vi "Main.vi"() -> ()   [LabVIEW 2013]
doc: "This template is for the Queued Message Handler design pattern.\n\nThe Event Handling Loop generates messages based on user interface actions.\n\nThe Message Handling Loop processes messages generated by the Event Handling Loop, or by other messages. The messages are string values, so new messages can be added easily to the Message Cases case structure in the Message Handling Loop. Each message cluster can also provide an optional value for Message Data, which is a variant that can be converted to whatever message-specific data is required."
uses:
  <vilib>/vision/Image Controls.llb/IMAQ Image.ctl
  Message Passing/MsgQ Loops enum.ctl
  Image Processing/Mask ROI FG Enum.ctl
  System Status/Status FG Enum.ctl
  Globals/Average Sector Data.vi
  controls/UI Data.ctl
  Message Queue/Message Queue.lvlib
  User Event - Stop/User Event - Stop.lvlib
  Image Processing/Image Processing.lvlib
  Common/State Machines/State Machine Lib.lvlib
  Message Passing/Main MsgQ.lvlib
  Common/GUI/GUI.lvlib
  <vilib>/rvi/interface/nirviReadWriteControl/nirviReadWriteControl.xnode
  FGs/FPGA_Reference.ctl
  FPGA Bitfiles/8-Tap-No-DRAM.lvbitx
  <vilib>/rvi/errors/niLvFpgaMergeErrorWithErrorCode.vi
  NiFpgaLv.dll
  <vilib>/rvi/errors/niLvFpgaAdjustHostInterfaceError.vi
panel:
  out "Analysis Ticks":u32
  out "Accumulate Ticks":u32
  out "FPGA Display Image":T1(plugin-control)
  out "Right Wingbeat Avg Graph":u8[](graph)
  in  "Start Serial Server":bool=TRUE
  out "Left Wingbeat Avg Graph":u8[](graph)
  in  "Stop Charts":bool
  in  "Wing ROIs":T2
  out "FPGA image info":T5={"Image Type"=0, "Unit"=enum."Undefined", "X Resolution"=2040, "Y Resolution"=1088, "X Step"=1.0, "Y Step"=1.0, "Image Name"="Image"} {"Image Type" items=["Grayscale (U8)", "Grayscale (I16)", "Grayscale (SGL)", "Complex (CSG)", "RGB (U32)", "HSL (U32)", "RGB (U64)", "Grayscale (U16)"]}
  in  "Stream?":bool
  out "FPGA Image":T1
  in  "Test Visual Response":bool
  in  "Test FPGA":bool
  out "Status Update":string="VI Stopped"
  in  "Define Mask":bool
  in  "Acquire Image":bool
  in  "Stop":bool
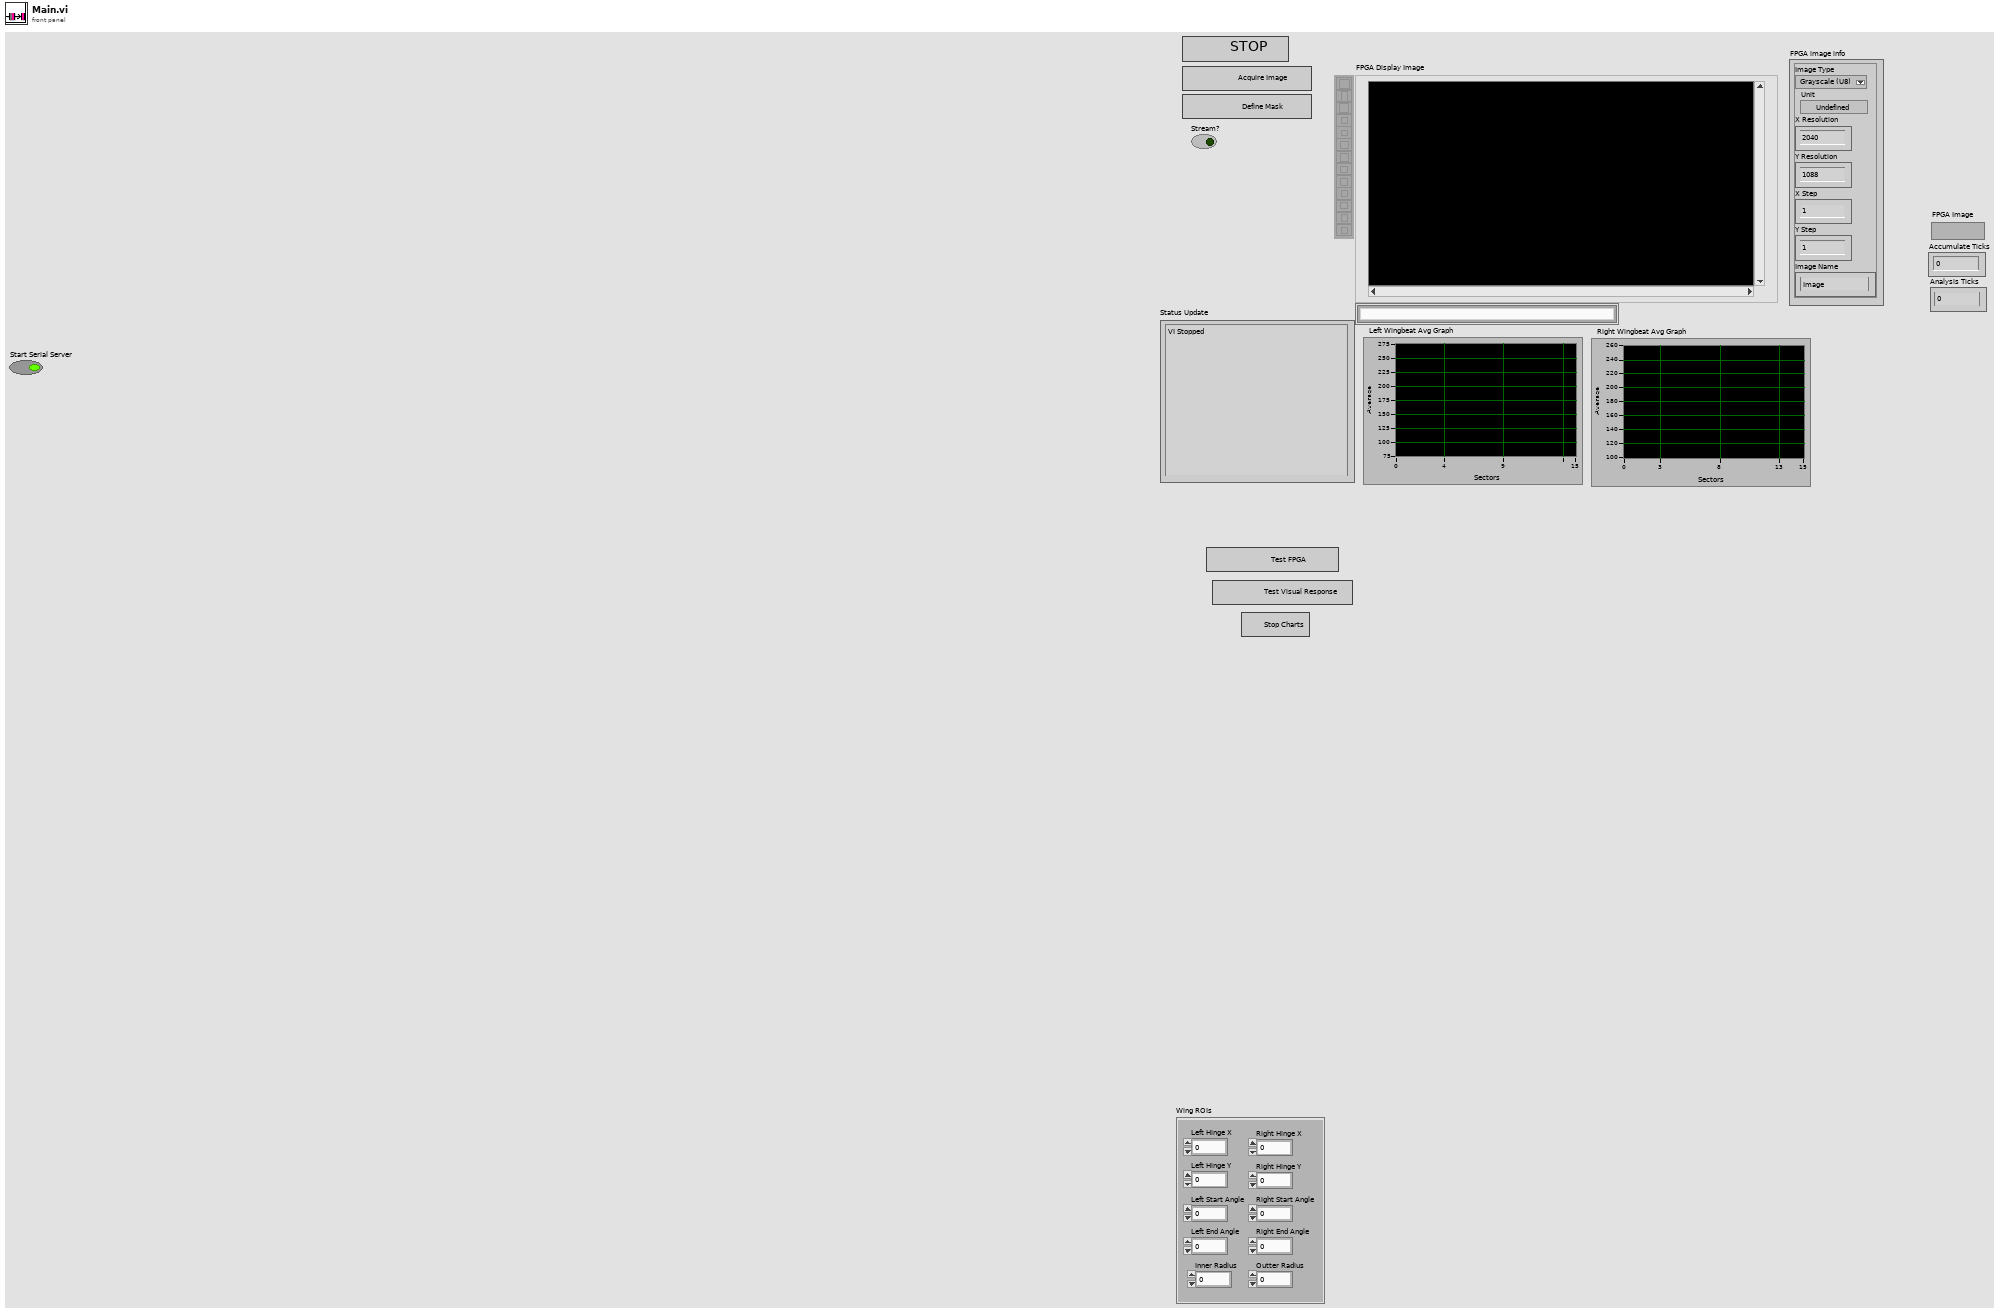
[diagram p1: front panel]
types:
  T1 = typedef "IMAQ Image.ctl" = refnum<image>
  T2 = cluster{"Left Hinge X":u16, "Left Hinge Y":u16, "Inner Radius":u16, "Outter Radius":u16, "Right Hinge X":u16, "Right Hinge Y":u16, "Right Start Angle":i16, "Right End Angle":i16, "Left Start Angle":i16, "Left End Angle":i16}
  T3 = typedef "Image Type" = u32
  T4 = typedef "Image Unit" = enum32{"Undefined", "Angström", "Micrometer", "Millimeter", "Centimeter", "Meter", "Kilometer", "Microinch", "Inch", "Feet", "Nautical miles", "Standard miles", "Steps"}
  T5 = cluster{"Image Type":T3, "Unit":T4, "X Resolution":i32, "Y Resolution":i32, "X Step":sgl, "Y Step":sgl, "Image Name":string}
  T6 = typedef "State Machine Lib.lvlib/STATE cluster.ctl" = cluster{"State":string, "Parameters":variant}
  T7 = typedef "Main MsgQ.lvlib/MsgQ Loops enum.ctl" = enum16{"User Interface", "Image Acq"}
  T8 = typedef "Status FG Enum.ctl" = enum16{"Reset", "Read", "Write"}
  T9 = typedef "Mask ROI FG Enum.ctl" = enum16{"Read", "Write"}
  T10 = typedef "FPGA_Reference.ctl" = refnum<k20>
  T11 = typedef "Mask ROI Cluster.ctl" = cluster{"left annulus":T12, "right annulus":T12, "Threshold Range":cluster{"Lower value":dbl, "Upper value":dbl}, "[Avg BG]":u8[], "Number of Sectors":u8, "Left ROI":T13, "Right ROI":T13, "Left Start Angle Duty Cycle":fxp<+,8,0>, "Left End Angle Duty Cycle":fxp<+,8,0>, "Right End Angle Duty Cycle":fxp<+,8,0>, "Right Start Angle Duty Cycle":fxp<+,8,0>, "[Sector ROIs]":T13[]}
  T12 = typedef "IMAQ Circle" = cluster{"Center X":i32, "Center Y":i32, "Inner Radius":i32, "Outer Radius":i32, "Start Angle":dbl, "End Angle":dbl}
  T13 = typedef "ROI Descriptor" = cluster{"Global Rectangle":i32[], "Contours":cluster{"ID":enum32{"External", "Internal"}, "Type":u32, "Coordinates":i32[]}[]}
  T14 = typedef "UI Data.ctl" = cluster{"Boolean <Replace Me>":bool, "Initial Message":string, "Numeric <Replace Me>":dbl, "Acquire Image Ref":refnum<vi>, "Define Mask Ref":refnum<vi>, "Status Update Ref":refnum<vi>, "Stop Button Ref":refnum<vi>, "FPGA Image":T1, "Processed Image":T1, "Left Annulus":cluster{"Center X":i32, "Center Y":i32, "Inner Radius":i32, "Outer Radius":i32, "Start Angle":dbl, "End Angle":dbl}, "Right Annulus":cluster{"Center X":i32, "Center Y":i32, "Inner Radius":i32, "Outer Radius":i32, "Start Angle":dbl, "End Angle":dbl}}
  T15 = typedef "Message Queue.lvlib/All Message Queues.ctl" = cluster{"UI":refnum<queue>}
  T16 = cluster{"Center X":i32, "Center Y":i32, "Inner Radius":i32, "Outer Radius":i32, "Start Angle":dbl, "End Angle":dbl}
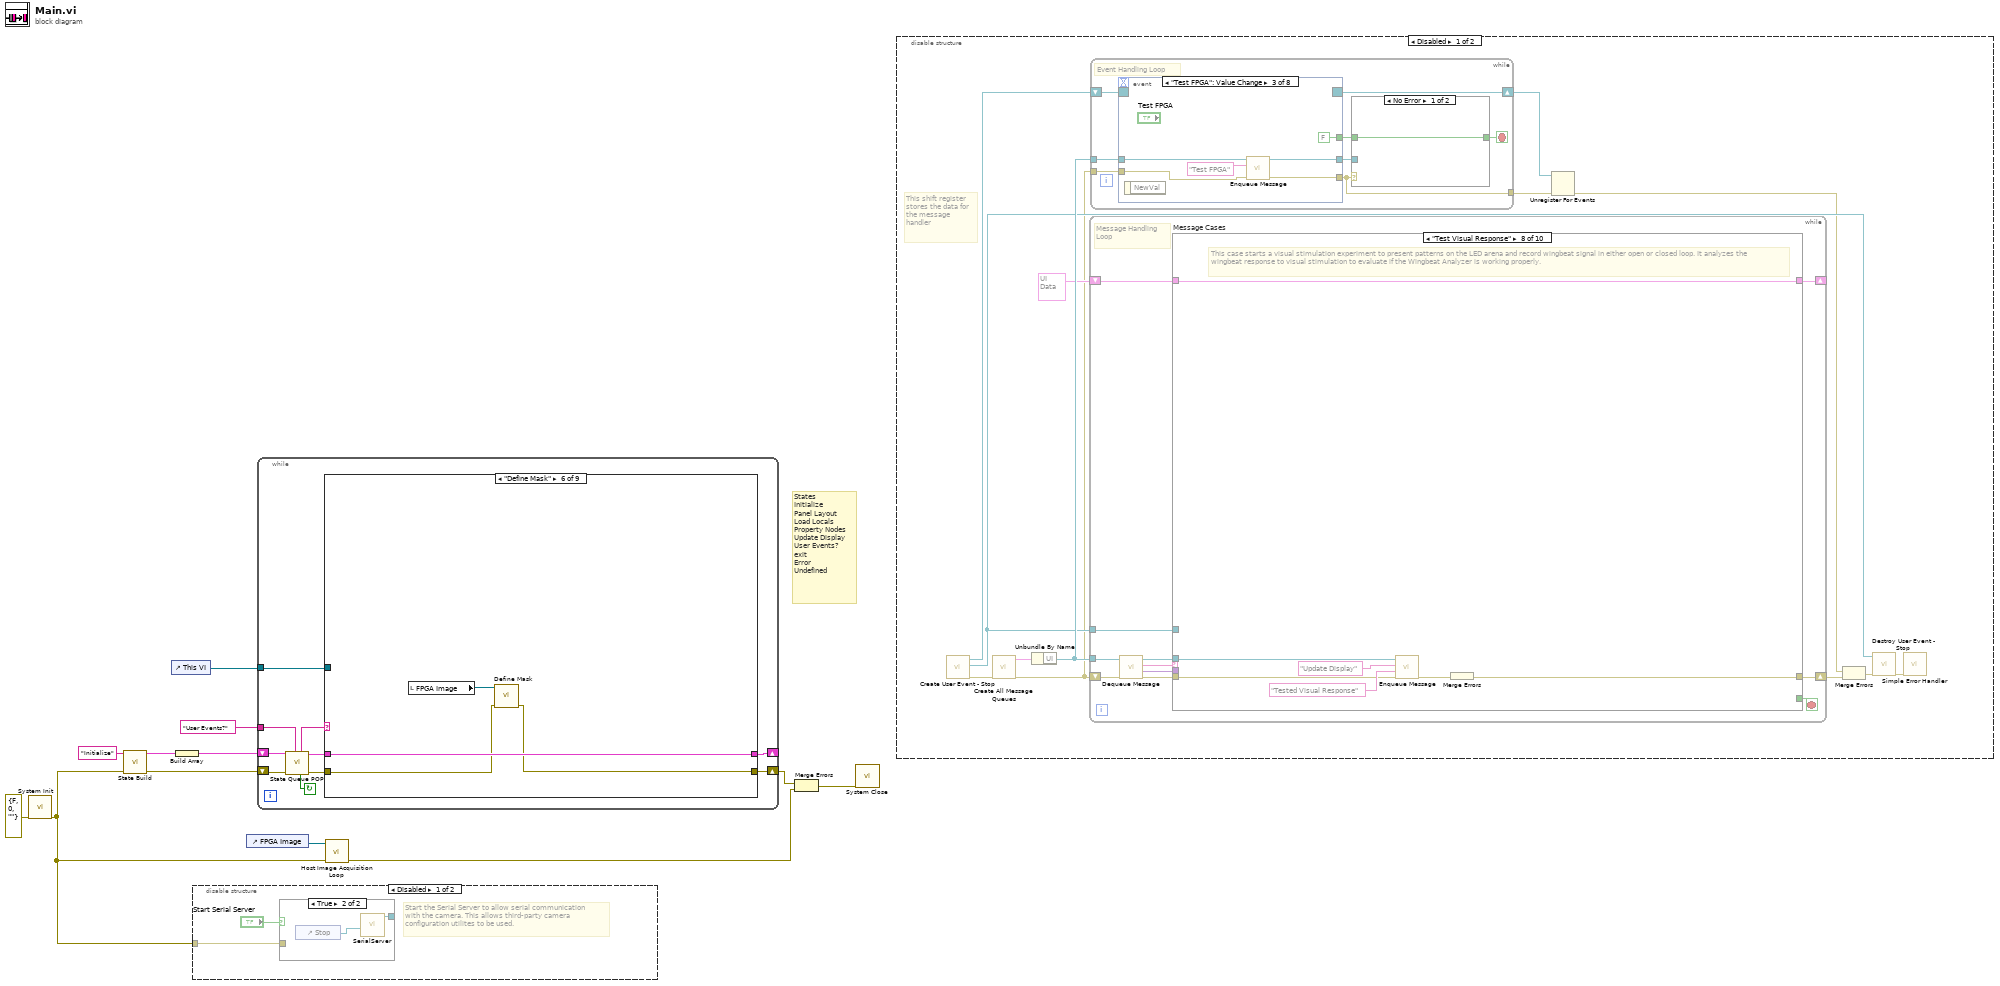
[diagram p0: block diagram]
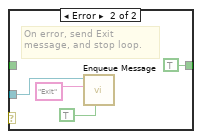
[diagram p4: hidden frame]
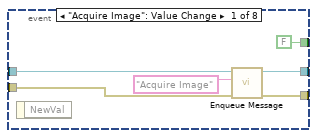
[diagram p5: hidden frame]
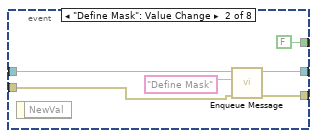
[diagram p6: hidden frame]
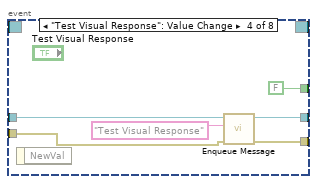
[diagram p7: hidden frame]
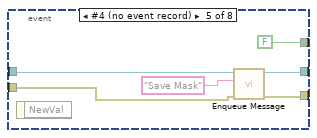
[diagram p8: hidden frame]
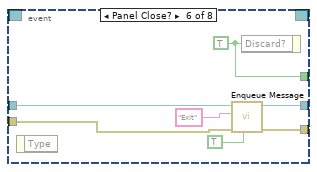
[diagram p9: hidden frame]
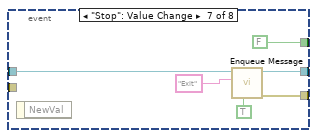
[diagram p10: hidden frame]
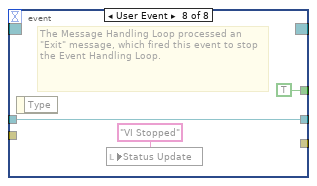
[diagram p11: hidden frame]
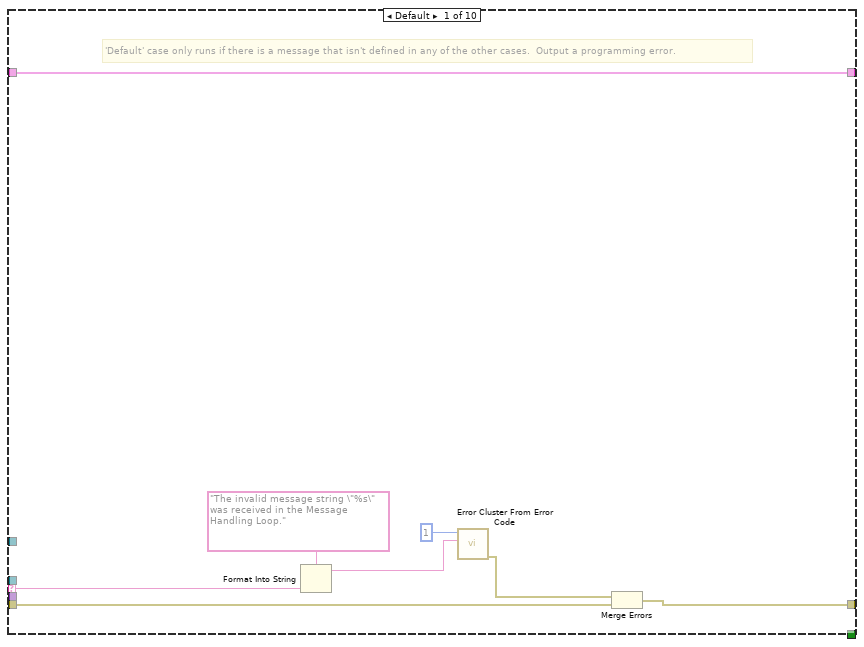
[diagram p12: hidden frame]
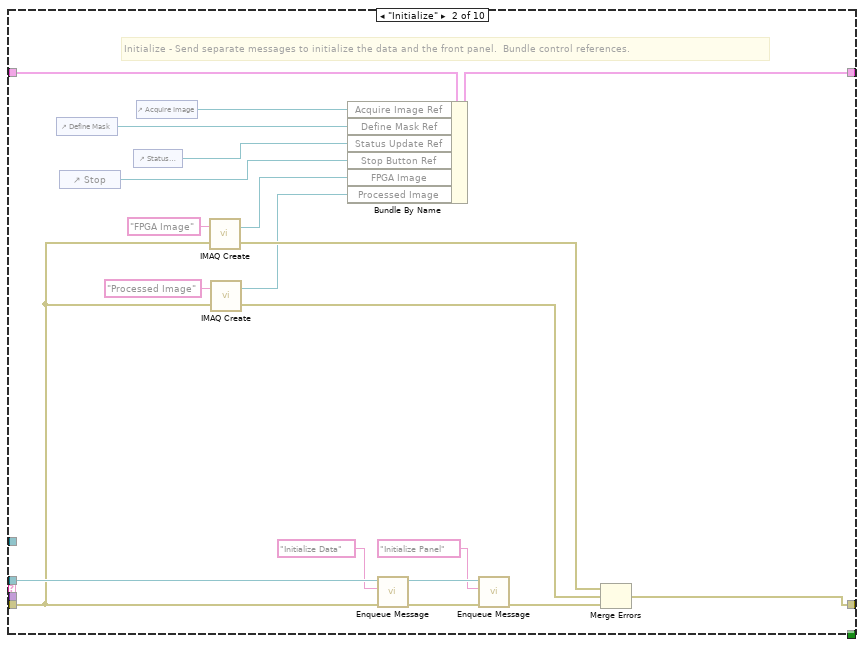
[diagram p13: hidden frame]
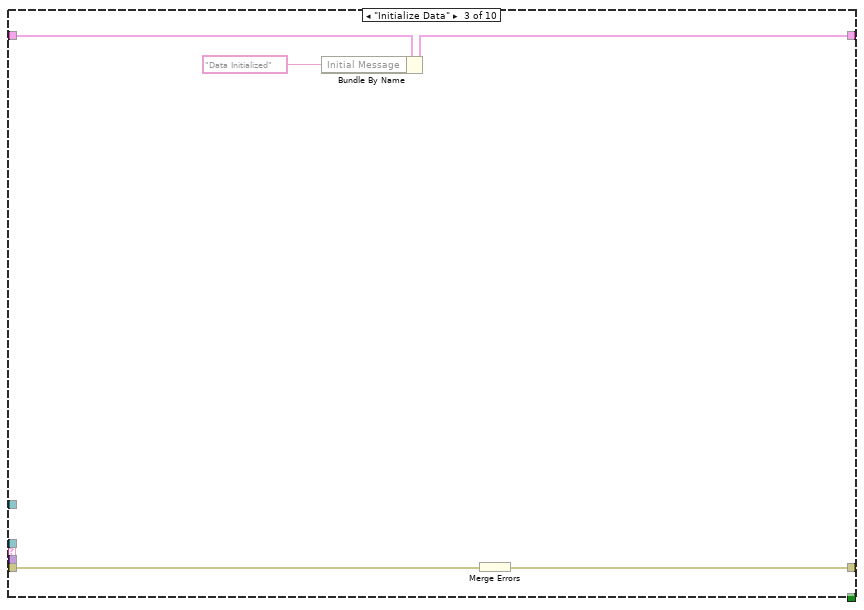
[diagram p14: hidden frame]
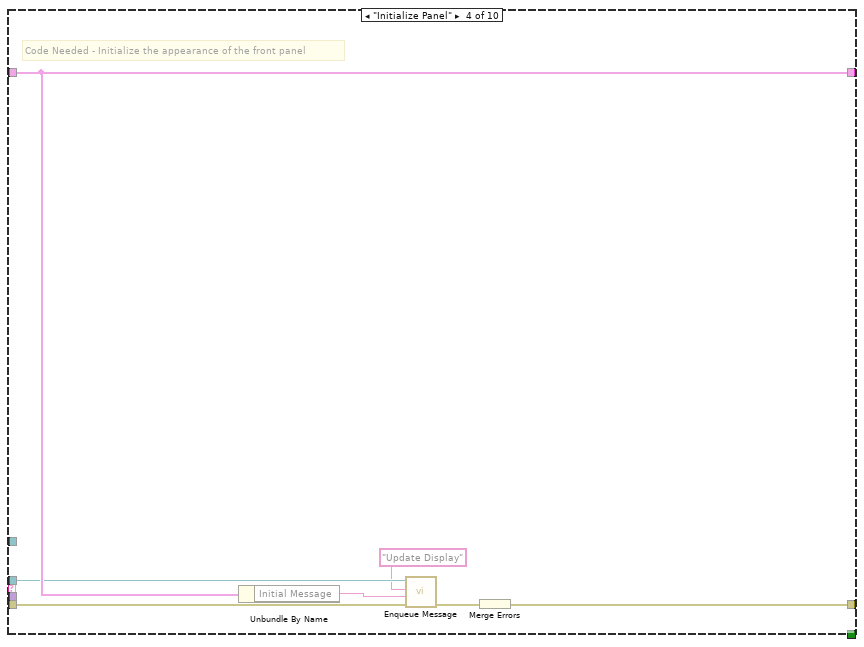
[diagram p15: hidden frame]
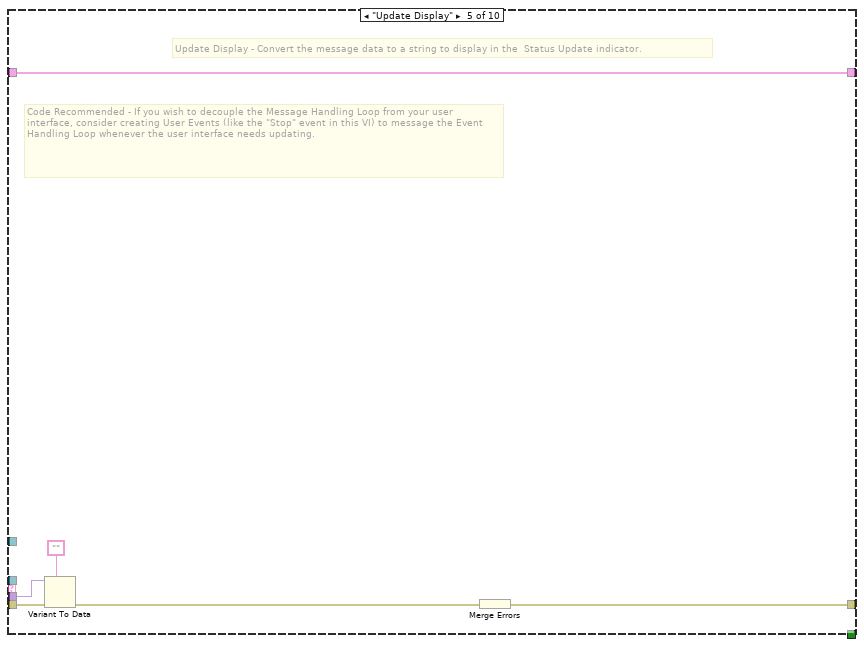
[diagram p16: hidden frame]
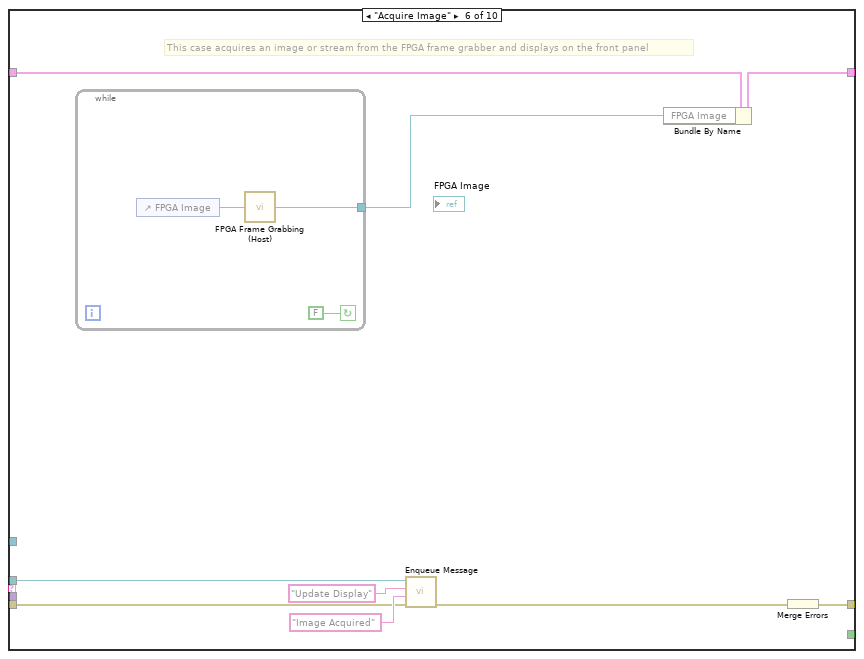
[diagram p17: hidden frame]
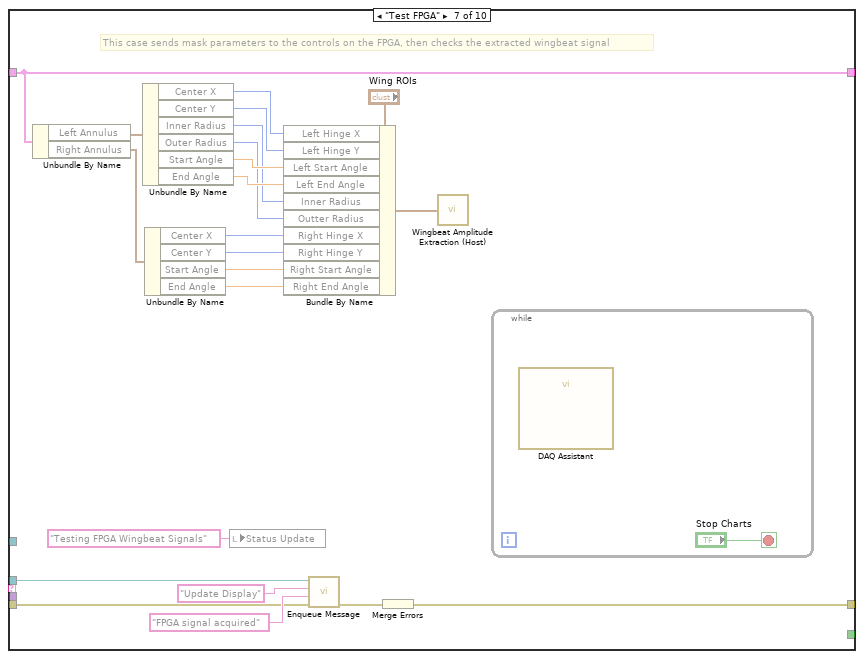
[diagram p18: hidden frame]
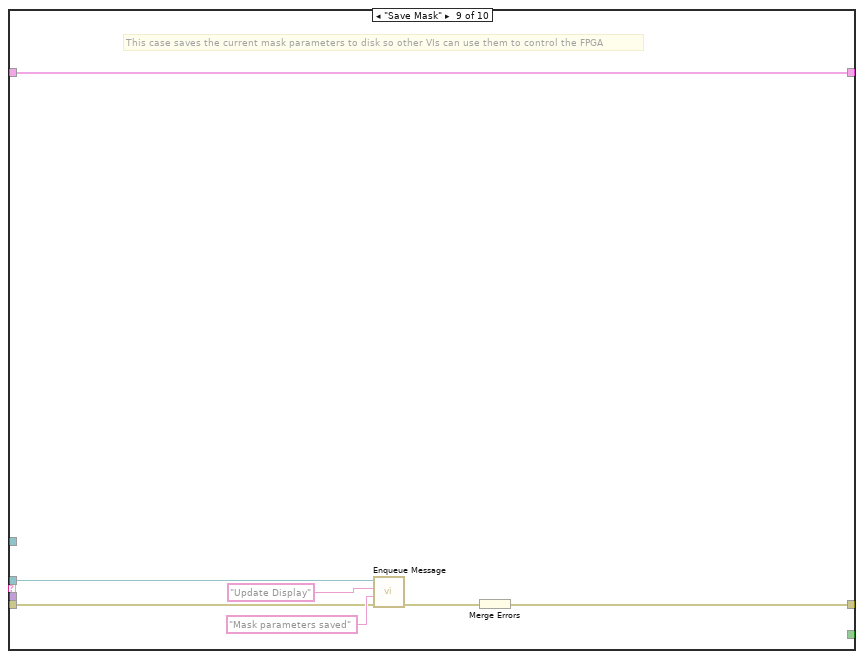
[diagram p19: hidden frame]
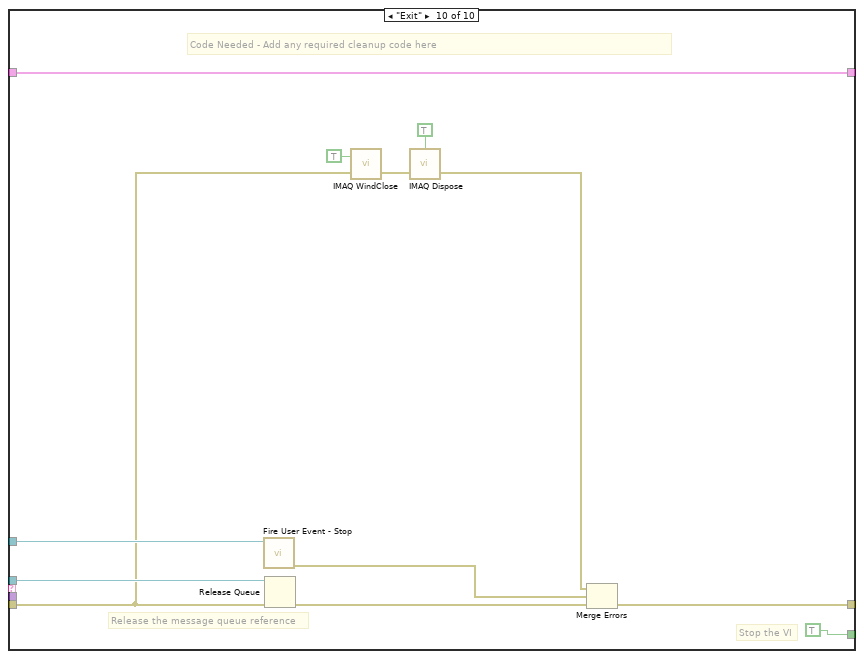
[diagram p20: hidden frame]
diagram:
  # "States\nInitialize\nPanel Layout\nLoad Locals\nProperty Nodes\nUpdate Display\nUser Events?\nexit\nError\nUndefined"
  n1 = call "System Init.vi"("error in (no error)"=errorcluster {"status"=FALSE, "code"=0, "source"=""}) -> ("error out"=w10:errorcluster)  [unwired: 10 in]
  n2 = call "State Build.vi"("error in (no error)"=w10, "State"="Initialize") -> ("error out"=w6:errorcluster, "State Out"=w8:T6)  [unwired: 8 in]
  n3 = control-ref of="This VI"() -> (w4:refnum<vi>)
  n4 = Build Array(w8) -> (w7:T6[])
  n5 = disable-structure shown="Disabled" {
    disable-tunnel: w10 -> [w13 _]
    frame Disabled {
      # "Start the Serial Server to allow serial communication\nwith the camera. This allows third-party camera\nconfiguration utilites to be used."
      n6 = case shown="True" "Start Serial Server" {
        tunnel: [_ w16] -> _
        tunnel: w13 -> [_ _]
        frame False {
        }
        frame True {
          n7 = control-ref of="Stop"() -> (w15:refnum<vi>)
          n8 = call "SerialServer.vi"("Stop Refnum"=w15) -> ("FPGA VI Reference Out"=w16:refnum<k20>)  [unwired: 6 in]
        }
      }
    }
    frame Enabled {
    }
  }
  n9 = control-ref of="FPGA Image"() -> (w12:refnum<vi>)
  n10 = while {
    shift-right: [w20] -> _
    shift-left: w7 -> [w26]
    shift-right: [w18] -> w3
    shift-left: w6 -> [w25]
    tunnel: "User Events?" ("State") -> [w23]
    tunnel: w4 -> [w21]
    stop <- w24 continue-if-true
    n11 = call "State Queue POP.vi"("Default state"=w23, "error in (no error)"=w25, "State que in"=w26) -> ("error out"=w17:errorcluster, "State que out"=w19:T6[], "Not Exit?"=w24:bool, "State case out"=w22:string)  [unwired: 4 in, 1 out]
    n12 = case shown="\"Define Mask\"" w22 {
      tunnel: w21 -> [_ _ w37 _ _ _ _ _ _]
      tunnel: [w28 w29 w34 w44 w46 w50 w54 w86 w112] -> w20
      tunnel: w19 -> [w28 w32 w34 w44 w46 w50 w53 _ w112]
      tunnel: [w27 w30 w35 w39 w45 w48 w52 w85 w110] -> w18
      tunnel: w17 -> [w27 w31 w36 w40 w45 w49 w51 w87 w94]
      frame Default {
      }
      frame "Initialize" {
        n13 = call "State Queue PUSH multiple states no parameters.vi"("States to queue"=string[] ["Panel Layout", "Load Locals", "Property Nodes", "Update Display"], "error in (no error)"=w31, "State que in"=w32) -> ("error out"=w30:errorcluster, "State que out"=w29:T6[])  [unwired: 7 in]
      }
      frame "Panel Layout" {
        # "Reset origin to 0,0"
        n14 = call "Reset all pane origins.vi"("error in (no error"=w36, "Vi Ref In"=w37) -> ("error out"=w35:errorcluster)  [unwired: 8 in, 1 out]
      }
      frame "Load Locals" {
        w41 = T3 0 items=["Grayscale (U8)", "Grayscale (I16)", "Grayscale (SGL)", "Complex (CSG)", "RGB (U32)", "HSL (U32)", "RGB (U64)", "Grayscale (U16)"] ("Image Type")
        n15 = call "IMAQ Create"("Image Name"="Display Image", "Image Type"=w41, "error in (no error)"=w40) -> ("New Image"=→"FPGA Display Image":T1, "error out"=w39:errorcluster)  [unwired: 2 in]
        n16 = local write "Stream?"(FALSE ("Stream?")) -> ()
      }
      frame "Property Nodes" {
      }
      frame "Define Mask" {
        n17 = local read "FPGA Image"() -> (w47:T1)
        n18 = call "Define Mask.vi"("error in (no error)"=w49, "FPGA Image"=w47) -> ("error out"=w48:errorcluster)  [unwired: 9 in]
      }
      frame "User Events?" {
        n19 = event shown="[0] Timeout" {
          selector: _ -> [_ _ _ _ _]
          dyn-events: _ -> [_ _ _ _ _]
          timeout: 200 -> [_ _ _ _ _]
          tunnel: [w57 w67 w70 w77 w80] -> w54
          tunnel: w53 -> [w58 w67 w70 w79 w83]
          tunnel: [w59 w64 w71 w76 w81] -> w52
          tunnel: w51 -> [w60 w65 w72 w78 w82]
          event Timeout {
            n20 = event-data() -> ()  [unwired: 1 in, 3 out]
            n21 = disable-structure shown="Enabled" {
              frame Disabled {
                n22 = call "FPGA Reference FG.vi"() -> ("FPGA VI Reference Out"=w63:T10)  [unwired: 11 in]
                n23 = xnode "Read/Write Control"("FPGA VI Reference In"=w63) -> ("Accumulate Ticks"=→"Accumulate Ticks", "Analysis Ticks"=→"Analysis Ticks":u32)  [unwired: 1 in, 2 out]
              }
              frame Enabled {
              }
            }
            n24 = call "State Queue PUSH.vi"("State case"="Update Display", "error in (no error)"=w60, "State que in"=w58) -> ("error out"=w59:errorcluster, "State que out"=w57:T6[])  [unwired: 7 in]
          }
          event "Acquire Image": Value Change {
            n25 = event-data() -> ()  [unwired: 1 in, 6 out]
            n26 = call "Send MsgQ.vi"("error in (no error)"=w65, "Message String"="Acquire Single Image", "Send to MsgQ"=MsgQ_Loops_enum."Image Acq") -> ("error out"=w64:errorcluster)  [unwired: 8 in]
          }
          event "Stream?": Value Change {
            n27 = event-data() -> ("NewVal"=w69:bool)  [unwired: 1 in, 5 out]
            n28 = call "Send MsgQ.vi"("error in (no error)"=w72, "Data In"=w69, "Message String"="Stream Image", "Send to MsgQ"=MsgQ_Loops_enum."Image Acq") -> ("error out"=w71:errorcluster)  [unwired: 7 in]
          }
          event "Define Mask": Value Change {
            n29 = event-data() -> ()  [unwired: 1 in, 6 out]
            n30 = call "State Queue PUSH.vi"("State case"="Define Mask", "error in (no error)"=w78, "State que in"=w79) -> ("error out"=w76:errorcluster, "State que out"=w77:T6[])  [unwired: 7 in]
          }
          event "Stop": Value Change {
            n31 = event-data() -> ()  [unwired: 1 in, 6 out]
            n32 = call "State Queue PUSH.vi"("State case"="exit", "error in (no error)"=w82, "State que in"=w83) -> ("error out"=w81:errorcluster, "State que out"=w80:T6[])  [unwired: 7 in]
          }
        }
      }
      frame "exit" {
        n33 = call "Broadcast Exit.vi"("error in"=w87) -> ("error out"=w85:errorcluster)  [unwired: 10 in]
        n34 = call "Queue EXIT state.vi"() -> ("Exit State Q"=w86:T6[])  [unwired: 1 in]
      }
      frame "Update Display" {
        n35 = local read "FPGA Image"() -> (w89:T1)
        n36 = local read "FPGA Display Image"() -> (w92:T1)
        n37 = call "Status FG.vi"("Operation"=Status_FG_Enum."Read") -> ("Status Out"=→"Status Update":string)  [unwired: 9 in, 1 out]
        n38 = call "Mask ROI FG.vi"("Operation"=Mask_ROI_FG_Enum."Read") -> ("Mask ROI Out"=w107:T11)  [unwired: 9 in, 1 out]
        n39 = Unbundle By Name(w107) -> ("Number of Sectors"=w104:u8)
        n40 = global read "Average Sector Data.vi" "[Average Sector Data]"() -> (w109:u8[])
        n41 = call "Overlay Image with Sector ROI.vi"("FPGA Display Image In"=w92, "error in"=w94, "FPGA Image"=w89) -> ("error out"=w93:errorcluster, "FPGA Display Image Out"=w88:T1)  [unwired: 7 in]
        n42 = call "IMAQ GetImageInfo"("error in (no error)"=w93, "Image"=w89) -> ("error out"=w111:errorcluster, "X Step"=w99:sgl, "Y Resolution"=w98:i32, "X Resolution"=w97:i32, "Y Step"=w100:sgl, "Unit"=w96:T4, "Image Name"=w101:string, "Image Type"=w95:T3)  [unwired: 2 in]
        n43 = Split 1D Array(array=w109, index=w104) -> (first subarray=→"Left Wingbeat Avg Graph":u8[], second subarray=→"Right Wingbeat Avg Graph":u8[])
        n44 = local write "FPGA Display Image"(w88) -> ()
        n45 = local read "FPGA image info"() -> (w103:T5)
        n46 = Bundle By Name(cluster=w103, "Image Type"=w95, "Unit"=w96, "X Resolution"=w97, "Y Resolution"=w98, "X Step"=w99, "Y Step"=w100, "Image Name"=w101) -> (→"FPGA image info":T5)
        n47 = call <vilib>:"Clear Errors.vi"("error in (no error)"=w111) -> ("error out"=w110:errorcluster)  [unwired: 6 in]
      }
    }
  }
  n48 = call "Host Image Acquisition Loop.vi"("error in"=w10, "Image Reference"=w12) -> ("error out"=w2:errorcluster)  [unwired: 9 in]
  n49 = Merge Errors(w3, w2) -> (w1:errorcluster)
  n50 = call "System Close.vi"("error in (no error)"=w1) -> ()  [unwired: 10 in, 1 out]
  n51 = disable-structure shown="Disabled" {
    frame Disabled {
      # "This shift register\nstores the data for the message handler"
      n52 = call "Create User Event - Stop.vi"() -> ("error out"=w121:errorcluster, "User Event - Stop"=w118:refnum<user-event>, "Stop Event Registration Refnum"=w122:refnum<event-registration>)  [unwired: 9 in]
      n53 = call "Create All Message Queues.vi"("error in (no error)"=w121) -> ("error out"=w113:errorcluster, "Message Queues out"=w125:T15)  [unwired: 9 in]
      n54 = Unbundle By Name(w125) -> ("UI"=w123:refnum<queue>)
      n55 = while {
        tunnel: w123 -> [w185]
        shift-right: [w194] -> _
        shift-left: T14 {"Boolean <Replace Me>"=TRUE, "Initial Message"="", "Numeric <Replace Me>"=0.0, "Acquire Image Ref"=refnum, "Define Mask Ref"=refnum, "Status Update Ref"=refnum, "Stop Button Ref"=refnum, "FPGA Image"=refnum, "Processed Image"=refnum, "Left Annulus"={"Center X"=0, "Center Y"=0, "Inner Radius"=0, "Outer Radius"=0, "Start Angle"=0.0, "End Angle"=0.0}, "Right Annulus"={"Center X"=0, "Center Y"=0, "Inner Radius"=0, "Outer Radius"=0, "Start Angle"=0.0, "End Angle"=0.0}} ("Data Cluster") -> [w195]
        tunnel: w118 -> [w191]
        shift-right: [w192] -> w124
        shift-left: w113 -> [w190]
        stop <- w193 stop-if-true
        # "Message Handling Loop"
        n56 = call "Dequeue Message.vi"("error in (no error)"=w190, "Message Queue"=w185) -> ("error out"=w189:errorcluster, "Message Data"=w187:variant, "Message"=w188:string, "dup Message Queue"=w186:refnum<queue>)  [unwired: 6 in]
        n57 = case "Message Cases" shown="\"Test Visual Response\"" w188 {
          selector: w188 -> [w201 _ _ _ _ _ _ _ _ _]
          tunnel: w186 -> [_ w221 _ w232 _ w249 w272 w280 w288 w304]
          tunnel: w189 -> [w198 w206 w228 w233 w240 w244 w273 w281 w286 w293]
          tunnel: [w196 w208 w224 w234 w241 w251 w271 w279 w291 w300] -> w192
          tunnel: w195 -> [w203 w218 w227 w235 w242 w246 w270 w285 w292 w303]
          tunnel: [w203 w217 w226 w235 w242 w245 w270 w285 w292 w303] -> w194
          tunnel: [_ _ _ _ _ _ _ _ _ TRUE] -> w193
          tunnel: w187 -> [_ _ _ _ w239 _ _ _ _ _]
          tunnel: w191 -> [_ _ _ _ _ _ _ _ _ w299]
          frame Default {
            # "'Default' case only runs if there is a message that isn't defined in any of the other cases.  Output a programming error."
            n58 = Format Into String(format string="The invalid message string \"%s\" was received in the Message Handling Loop." ("Unknown Message Error Text"), w201) -> (resulting string=w199:string)  [unwired: 2 in, 1 out]
            n59 = call <vilib>:"Error Cluster From Error Code.vi"("error message (\"\")"=w199, "error code (0)"=1) -> ("error out"=w197:errorcluster)  [unwired: 7 in]
            n60 = Merge Errors(w197, w198) -> (w196:errorcluster)
          }
          frame "Initialize" {
            # "Initialize - Send separate messages to initialize the data and the front panel.  Bundle control references."
            n61 = control-ref of="Define Mask"() -> (w215:refnum<vi>)
            n62 = control-ref of="Stop"() -> (w213:refnum<vi>)
            n63 = control-ref of="Status Update"() -> (w214:refnum<vi>)
            n64 = control-ref of="Acquire Image"() -> (w216:refnum<vi>)
            n65 = call "IMAQ Create"("Image Name"="FPGA Image", "error in (no error)"=w206) -> ("New Image"=w211:T1, "error out"=w207:errorcluster)  [unwired: 3 in]
            n66 = call "IMAQ Create"("Image Name"="Processed Image", "error in (no error)"=w206) -> ("New Image"=w204:T1, "error out"=w205:errorcluster)  [unwired: 3 in]
            n67 = Bundle By Name(cluster=w218, "Acquire Image Ref"=w216, "Define Mask Ref"=w215, "Status Update Ref"=w214, "Stop Button Ref"=w213, "FPGA Image"=w211, "Processed Image"=w204) -> (w217:T14)
            n68 = call "Enqueue Message.vi"("error in (no error)"=w206, "Message"="Initialize Data", "Message Queue"=w221) -> ("error out"=w223:errorcluster, "dup Message Queue"=w222:refnum<queue>)  [unwired: 7 in]
            n69 = call "Enqueue Message.vi"("error in (no error)"=w223, "Message"="Initialize Panel", "Message Queue"=w222) -> ("error out"=w209:errorcluster)  [unwired: 7 in, 1 out]
            n70 = Merge Errors(w207, w205, w209) -> (w208:errorcluster)
          }
          frame "Initialize Data" {
            n71 = Bundle By Name(cluster=w227, "Initial Message"="Data Initialized") -> (w226:T14)
            n72 = Merge Errors(w228) -> (w224:errorcluster)
          }
          frame "Initialize Panel" {
            # "Code Needed - Initialize the appearance of the front panel"
            n73 = Unbundle By Name(w235) -> ("Initial Message"=w229:string)
            n74 = call "Enqueue Message.vi"("error in (no error)"=w233, "Message Data"=w229, "Message"="Update Display", "Message Queue"=w232) -> ("error out"=w231:errorcluster)  [unwired: 6 in, 1 out]
            n75 = Merge Errors(w231) -> (w234:errorcluster)
          }
          frame "Update Display" {
            # "Code Recommended - If you wish to decouple the Message Handling Loop from your user interface, consider creating User Events (like the \"Stop\" event in this VI) to message the Event Handling Loop whenever the user interface needs updating."
            # "Update Display - Convert the message data to a string to display in the  Status Update indicator."
            n76 = Variant To Data(error in=w240, type="", Variant=w239) -> (data=w236:string, error out=w237:errorcluster)
            n77 = Merge Errors(w237) -> (w241:errorcluster)
          }
          frame "Acquire Image" {
            # "This case acquires an image or stream from the FPGA frame grabber and displays on the front panel"
            n78 = while {
              tunnel: [w254] -> w243
              stop <- FALSE continue-if-true
              n79 = control-ref of="FPGA Image"() -> (w253:refnum<vi>)
              n80 = call "FPGA Frame Grabbing (Host).vi"("Ctl Refnum"=w253) -> ("Image"=w254:T1)
            }
            n81 = call "Enqueue Message.vi"("error in (no error)"=w244, "Message Data"="Image Acquired" ("\"Do Something\" button pressed"), "Message"="Update Display", "Message Queue"=w249) -> ("error out"=w250:errorcluster)  [unwired: 6 in, 1 out]
            n82 = Bundle By Name(cluster=w246, "FPGA Image"=w243) -> (w245:T14)
            n83 = Merge Errors(w250) -> (w251:errorcluster)
          }
          frame "Test FPGA" {
            # "This case sends mask parameters to the controls on the FPGA, then checks the extracted wingbeat signal"
            n84 = Unbundle By Name(w270) -> ("Left Annulus"=w269:T16, "Right Annulus"=w268:T16)
            n85 = Unbundle By Name(w269) -> ("Center X"=w266:i32, "Center Y"=w265:i32, "Inner Radius"=w262:i32, "Outer Radius"=w261:i32, "Start Angle"=w264:dbl, "End Angle"=w263:dbl)
            n86 = Unbundle By Name(w268) -> ("Center X"=w260:i32, "Center Y"=w259:i32, "Start Angle"=w258:dbl, "End Angle"=w257:dbl)
            n87 = local write "Status Update"("Testing FPGA Wingbeat Signals" ("Status Update")) -> ()
            n88 = Bundle By Name(cluster="Wing ROIs", "Left Hinge X"=w266, "Left Hinge Y"=w265, "Left Start Angle"=w264, "Left End Angle"=w263, "Inner Radius"=w262, "Outter Radius"=w261, "Right Hinge X"=w260, "Right Hinge Y"=w259, "Right Start Angle"=w258, "Right End Angle"=w257) -> (w256:T2)
            n89 = call "Enqueue Message.vi"("error in (no error)"=w273, "Message Data"="FPGA signal acquired" ("\"Do Something\" button pressed"), "Message"="Update Display", "Message Queue"=w272) -> ("error out"=w276:errorcluster)  [unwired: 6 in, 1 out]
            n90 = Merge Errors(w276) -> (w271:errorcluster)
            n91 = call "Wingbeat Amplitude Extraction (Host).vi"("Wing ROIs"=w256) -> ()  [unwired: 1 in]
            n92 = while {
              stop <- "Stop Charts" stop-if-true
              n93 = call "DAQ Assistant"() -> ("data"=w277:dynamicdata)  [unwired: 17 in, 2 out]
            }
          }
          frame "Test Visual Response" {
            # "This case starts a visual stimulation experiment to present patterns on the LED arena and record wingbeat signal in either open or closed loop. It analyzes the wingbeat response to visual stimulation to evaluate if the Wingbeat Analyzer is working properly."
            n94 = call "Enqueue Message.vi"("error in (no error)"=w281, "Message Data"="Tested Visual Response" ("\"Do Something\" button pressed"), "Message"="Update Display", "Message Queue"=w280) -> ("error out"=w284:errorcluster)  [unwired: 6 in, 1 out]
            n95 = Merge Errors(w284) -> (w279:errorcluster)
          }
          frame "Save Mask" {
            # "This case saves the current mask parameters to disk so other VIs can use them to control the FPGA"
            n96 = call "Enqueue Message.vi"("error in (no error)"=w286, "Message Data"="Mask parameters saved" ("\"Do Something Else\" button pressed"), "Message"="Update Display", "Message Queue"=w288) -> ("error out"=w287:errorcluster)  [unwired: 6 in, 1 out]
            n97 = Merge Errors(w287) -> (w291:errorcluster)
          }
          frame "Exit" {
            # "Stop the VI"
            # "Release the message queue reference"
            # "Code Needed - Add any required cleanup code here"
            n98 = call "Fire User Event - Stop.vi"("User Event - Stop"=w299) -> ("error out"=w298:errorcluster)  [unwired: 10 in]
            n99 = Release Queue(queue=w304, error in (no error)=w293) -> (error out=w301:errorcluster)  [unwired: 1 in, 2 out]
            n100 = call "IMAQ WindClose"("Close All Windows (False)"=TRUE, "error in (no error)"=w293) -> ("error out"=w295:errorcluster)  [unwired: 4 in]
            n101 = call "IMAQ Dispose"("All Images? (No)"=TRUE, "error in (no error)"=w295) -> ("error out"=w294:errorcluster)  [unwired: 4 in]
            n102 = Merge Errors(w294, w298, w301) -> (w300:errorcluster)
          }
        }
      }
      n103 = while {
        tunnel: w123 -> [w133]
        tunnel: [w129] -> w116
        shift-right: [w127] -> w115
        shift-left: w122 -> [w128]
        tunnel: w113 -> [w126]
        stop <- w131 stop-if-true
        # "Event Handling Loop"
        n104 = event shown="[2] \"Test FPGA\": Value Change" {
          selector: w128 -> [_ _ _ _ _ _ _ _]
          dyn-events: [_ _ _ _ _ _ _ _] -> w127
          timeout: _ -> [_ _ _ _ _ _ _ _]
          tunnel: [FALSE ("Discard?") FALSE ("Discard?") FALSE ("Discard?") FALSE ("Discard?") FALSE ("Discard?") w175 FALSE ("Discard?") TRUE ("Discard?")] -> w132
          tunnel: w133 -> [w144 w150 w156 w161 w166 w174 w181 w184]
          tunnel: [w143 w148 w153 w158 w163 w173 w180 _] -> w129
          tunnel: [w142 w149 w152 w160 w165 w172 w178 w184] -> w130
          tunnel: w126 -> [w140 w146 w154 w157 w164 w169 _ _]
          event "Acquire Image": Value Change {
            n105 = event-data() -> ()  [unwired: 1 in, 1 out]
            n106 = call "Enqueue Message.vi"("error in (no error)"=w140, "Message"="Acquire Image", "Message Queue"=w144) -> ("error out"=w143:errorcluster, "dup Message Queue"=w142:refnum<queue>)  [unwired: 7 in]
          }
          event "Define Mask": Value Change {
            n107 = event-data() -> ()  [unwired: 1 in, 1 out]
            n108 = call "Enqueue Message.vi"("error in (no error)"=w146, "Message"="Define Mask", "Message Queue"=w150) -> ("error out"=w148:errorcluster, "dup Message Queue"=w149:refnum<queue>)  [unwired: 7 in]
          }
          event "Test FPGA": Value Change {
            n109 = event-data() -> ()  [unwired: 1 in, 1 out]
            n110 = call "Enqueue Message.vi"("error in (no error)"=w154, "Message"="Test FPGA", "Message Queue"=w156) -> ("error out"=w153:errorcluster, "dup Message Queue"=w152:refnum<queue>)  [unwired: 7 in]
          }
          event "Test Visual Response": Value Change {
            n111 = event-data() -> ()  [unwired: 1 in, 1 out]
            n112 = call "Enqueue Message.vi"("error in (no error)"=w157, "Message"="Test Visual Response", "Message Queue"=w161) -> ("error out"=w158:errorcluster, "dup Message Queue"=w160:refnum<queue>)  [unwired: 7 in]
          }
          event #4 (no event record) {
            n113 = event-data() -> ()  [unwired: 1 in, 1 out]
            n114 = call "Enqueue Message.vi"("error in (no error)"=w164, "Message"="Save Mask", "Message Queue"=w166) -> ("error out"=w163:errorcluster, "dup Message Queue"=w165:refnum<queue>)  [unwired: 7 in]
          }
          event Panel Close? {
            w175 = TRUE ("Discard?")
            n115 = event-data() -> ()  [unwired: 1 in, 1 out]
            n116 = call "Enqueue Message.vi"("Priority Message? (F)"=TRUE, "error in (no error)"=w169, "Message"="Exit", "Message Queue"=w174) -> ("error out"=w173:errorcluster, "dup Message Queue"=w172:refnum<queue>)  [unwired: 6 in]
            n117 = event-data("Discard?"=w175) -> ()  [unwired: 1 in, 1 out]
          }
          event "Stop": Value Change {
            n118 = event-data() -> ()  [unwired: 1 in, 1 out]
            n119 = call "Enqueue Message.vi"("Priority Message? (F)"=TRUE, "Message"="Exit", "Message Queue"=w181) -> ("error out"=w180:errorcluster, "dup Message Queue"=w178:refnum<queue>)  [unwired: 7 in]
          }
          event User Event {
            # "The Message Handling Loop processed an \"Exit\" message, which fired this event to stop the Event Handling Loop."
            n120 = event-data() -> ()  [unwired: 1 in, 1 out]
            n121 = local write "Status Update"("VI Stopped" ("VI Stopped")) -> ()
          }
        }
        n122 = case shown="No Error" w129 {
          tunnel: [w134 TRUE ("Discard?")] -> w131
          tunnel: w132 -> [w134 _]
          tunnel: w130 -> [_ w137]
          frame No Error {
          }
          frame Error {
            # "On error, send Exit message, and stop loop."
            n123 = call "Enqueue Message.vi"("Priority Message? (F)"=TRUE, "Message"="Exit", "Message Queue"=w137) -> ()  [unwired: 7 in, 2 out]
          }
        }
      }
      n124 = Unregister For Events(event registration refnum=w115, error in=w116) -> (error out=w117:errorcluster)
      n125 = Merge Errors(w117, w124) -> (w119:errorcluster)
      n126 = call "Destroy User Event - Stop.vi"("error in (no error)"=w119, "User Event - Stop"=w118) -> ("error out"=w120:errorcluster)  [unwired: 9 in]
      n127 = call <vilib>:"Simple Error Handler.vi"("error in (no error)"=w120) -> ()  [unwired: 4 in, 5 out]
    }
    frame Enabled {
    }
  }
